vi "Set-Exposure-time.vi"(7 "Camera":u32, 8 "error in (no error)":errorcluster, 10 "Acquis. params. ref. in":refnum<data-value>, 11 "Camera in":refnum<class "Camera.lvclass">) -> (0 "error out":errorcluster, 1 "Exposure time":dbl caption="Exposure time [s]", 2 "Acquis. params. ref.":refnum<data-value>, 3 "Camera out":refnum<class "Camera.lvclass">)   [LabVIEW 2013, in "CameraVision.lvlib" / "Camera.lvclass"]
uses:
  Camera.lvclass
  Main/Acquisition/CV-Acquisition.lvclass
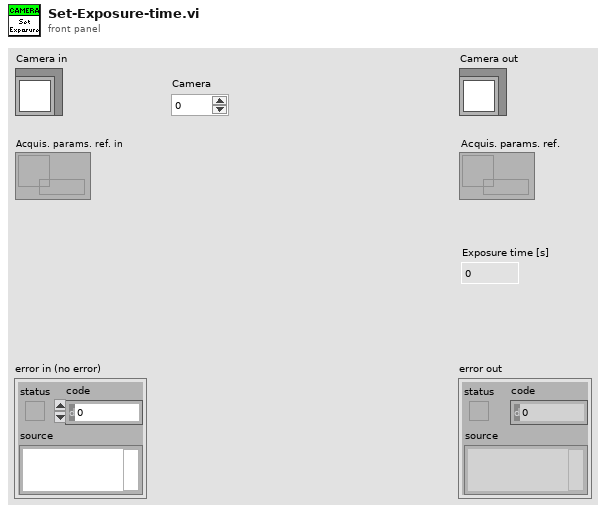
[diagram p1: front panel]
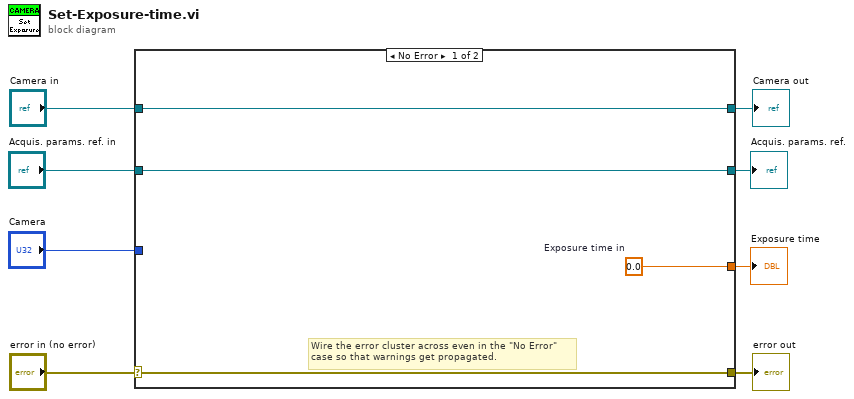
[diagram p0: block diagram]
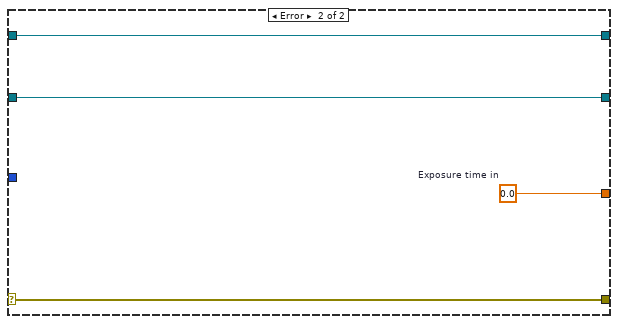
[diagram p2: hidden frame]
diagram:
  n1 = case shown="No Error" "error in (no error)" {
    selector: "error in (no error)" -> [w11 w16]
    tunnel: [w11 w16] -> w7
    tunnel: [w12 w15] -> w5
    tunnel: "Camera in" -> [w12 w15]
    tunnel: [w9 w13] -> w4
    tunnel: "Acquis. params. ref. in" -> [w10 w14]
    tunnel: [w10 w14] -> w2
    tunnel: "Camera" -> [_ _]
    frame No Error {
      w9 = 0.0  # Exposure time in
      # "Wire the error cluster across even in the \"No Error\"\ncase so that warnings get propagated."
    }
    frame Error {
      w13 = 0.0  # Exposure time in
    }
  }
  "error out" <- w7
  "Camera out" <- w5
  "Exposure time" <- w4
  "Acquis. params. ref." <- w2
